vi "Get Item Symbles in Project.vi"(8 "error in (no error)":errorcluster caption="错误输入（无错误）", 11 "Device Tree Ref":refnum<vi>) -> (0 "error out":errorcluster caption="错误输出")   [LabVIEW 2013]
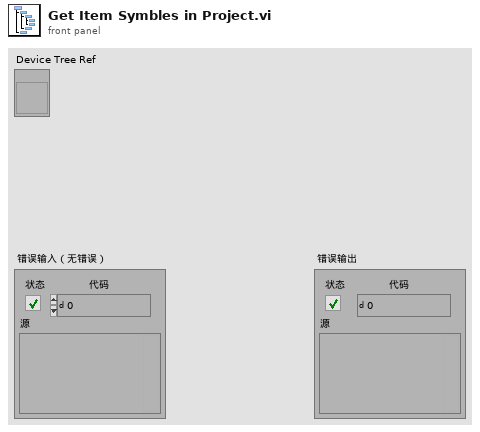
[diagram p1: front panel]
types:
  T1 = enum32{"None", "LabVIEW", "Mac OS", "Windows", "Default"}
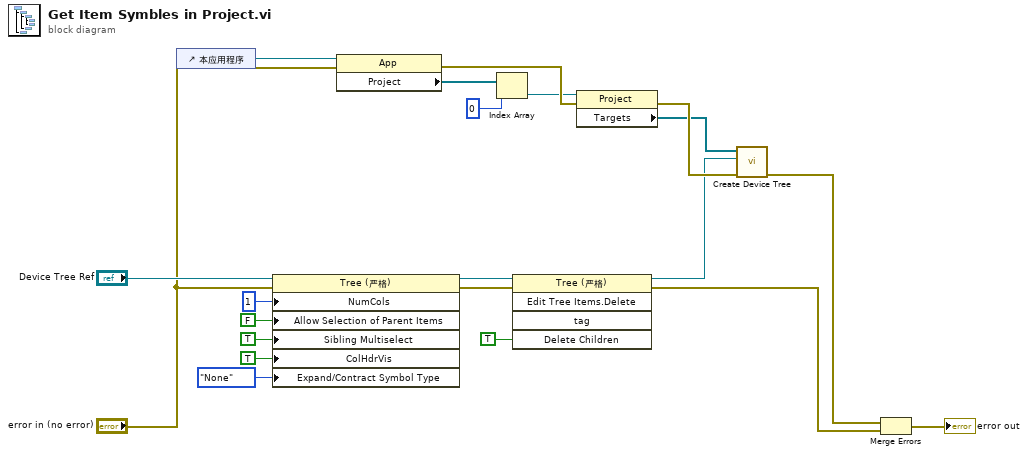
[diagram p0: block diagram]
diagram:
  n1 = control-ref of="本应用程序"() -> (w14:refnum<vi>)
  n2 = property class="Tree (严格)"(reference="Device Tree Ref", error in="error in (no error)", "NumCols"=u32 1 ("列数"), "Allow Selection of Parent Items"=FALSE ("允许选择父项"), "Sibling Multiselect"=TRUE ("同辈多选"), "ColHdrVis"=TRUE ("允许选择父项"), "Expand/Contract Symbol Type"=T1."None" ("缩进/移出符号:符号类型")) -> (reference out=w8:refnum<vi>, error out=w7:errorcluster)
  n3 = property class="App"(reference=w14, error in="error in (no error)") -> (error out=w19:errorcluster, "Project"=w20:refnum<vi>[])  [unwired: 1 out]
  n4 = Index Array(array=w20, index=0 ("索引")) -> (element=w18:refnum<vi>)
  n5 = invoke class="Tree (严格)" method="Edit Tree Items.Delete"(reference=w8, error in=w7, "Delete Children"=TRUE ("删除子项？")) -> (reference out=w5:refnum<vi>, error out=w1:errorcluster)  [unwired: 2 in, 3 out]
  n6 = property class="Project"(reference=w18, error in=w19) -> (error out=w17:errorcluster, "Targets"=w13:refnum<vi>[])  [unwired: 1 out]
  n7 = call "Create Device Tree.vi"("error in (no error)"=w17, "Tree Control Ref"=w5, "Project Item Array"=w13) -> ("error out"=w16:errorcluster)  [unwired: 8 in]
  n8 = Merge Errors(w16, w1) -> (→"error out":errorcluster)
